vi "autoslice_delta_z_fixed.vi"() -> ()   [LabVIEW 2021]
panel:
  in  "Non moving mode":bool
  in  "System state during slices":string(combo)="Continuous imaging"
  in  "pulse duration (T/2)":dbl=0.0005 format="%#_13p"
  in  "Motor speed":string(combo)="Full step"
  in  "Use predefined list":bool
  in  "Predefined pulse steps":i32[](array[numeric])=[127, 63, 62, 58, 56, -72, -104, 24, 8, 72, 73, 77, 79, 15, 47, -81, -65, -97, 31, 29, 28, 92, 76, 12, 4, 36, -92, -90, -89, -121, -105, -41, -33, -49, -113, -114, 14, 46, 38, 6, 2, 18, 82, 83, -45, -61, -53, -21, -17, -25, -57, 71, 7, 23, 19, 3, 1, 9, 41, -87, -23, -31, -27, -11, -9, -13, -29, -93, -125, -117, -119, -127, -128, -124, -108, -44, -12, -16, -14, -6, -5, -7, -15, -47, -63, -59, -60, -64, 64, 66, 74, 106, 122, 120, 121, 125, -3, -4, -8, -24, -32, -30, 98, 96, 32, 33, 37, 53, 61, 60, -68, -66, -2, 126, 124, 116, 112, 113, 49, 48, 16, -112, -110, -102, -98, 30, 94, 95] format="%.0p"
  in  "milliseconds to wait after bed move":u32=500
  in  "milliseconds to wait after imaging ends":u32=500
  in  "pulses to move (delta z)":i32=20
  out "pulses moving":i32=20
  out "Wait for imaging":bool
  out "Wait for move":bool
  in  "max runs":i32=6 min=2 step=2
  out "Current run":i32=6
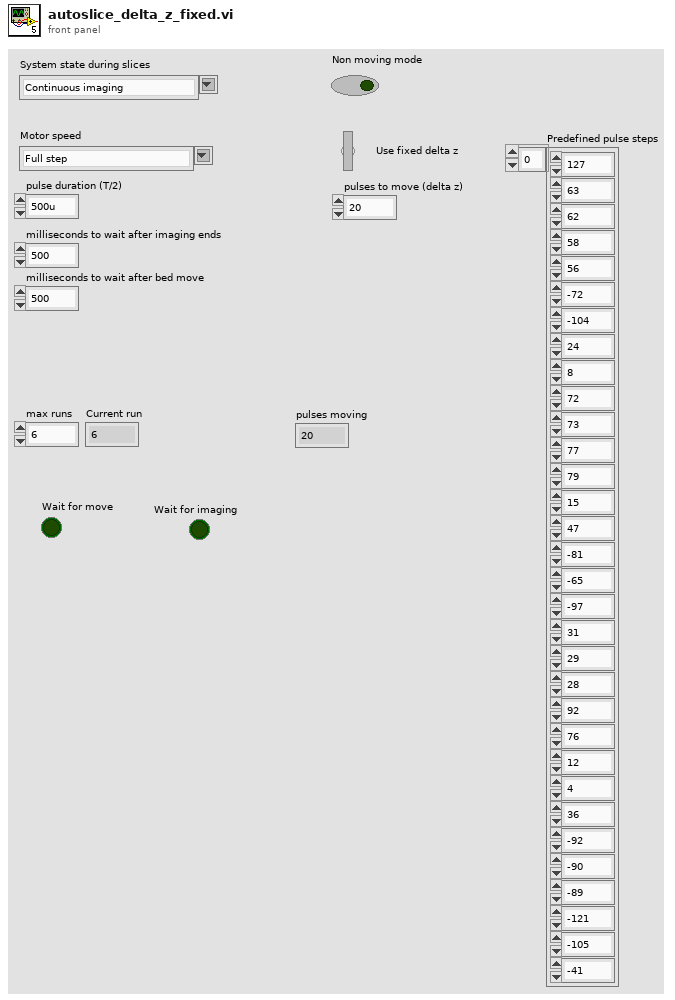
[diagram p1: front panel]
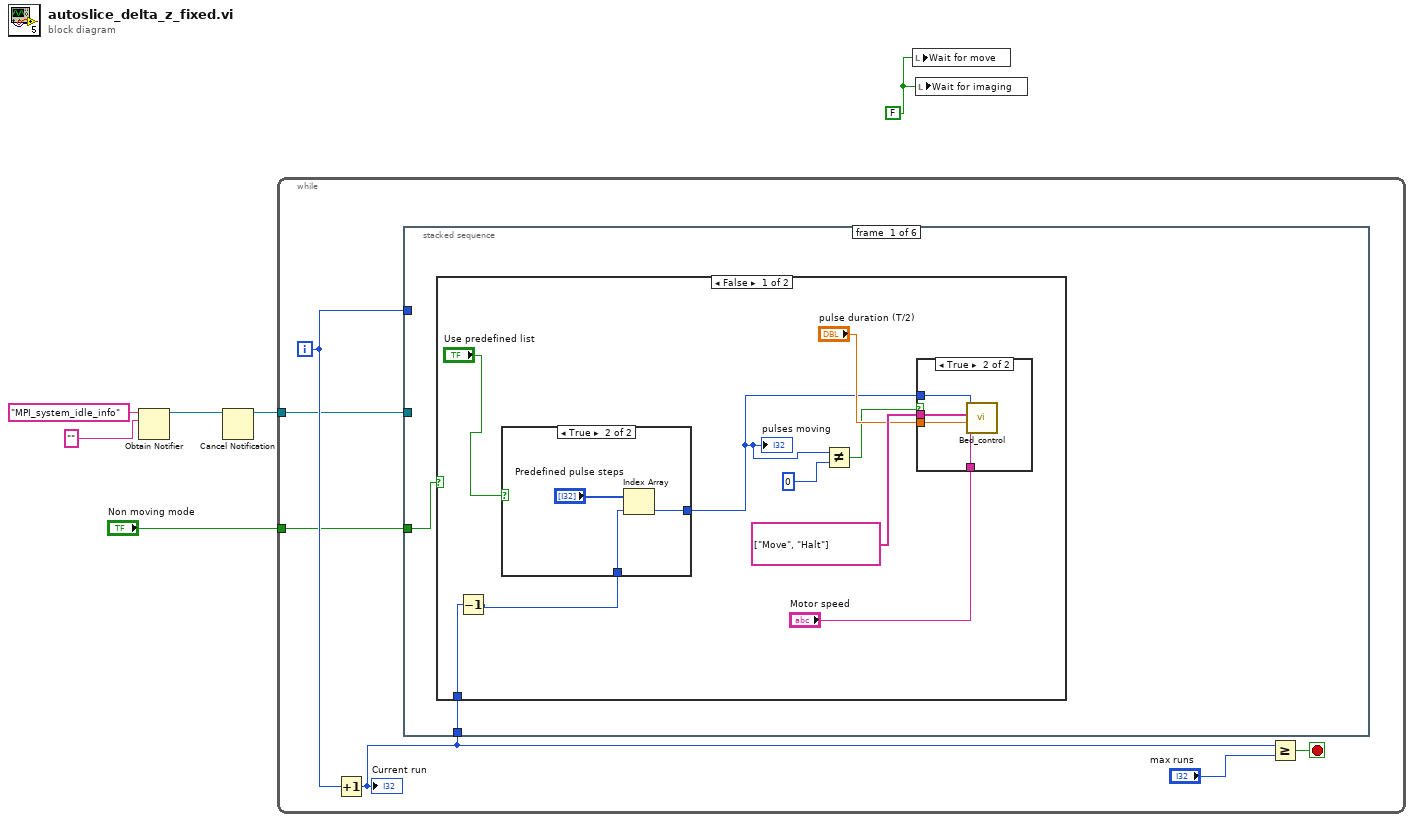
[diagram p0: block diagram]
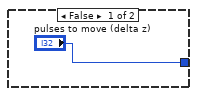
[diagram p3: hidden frame]
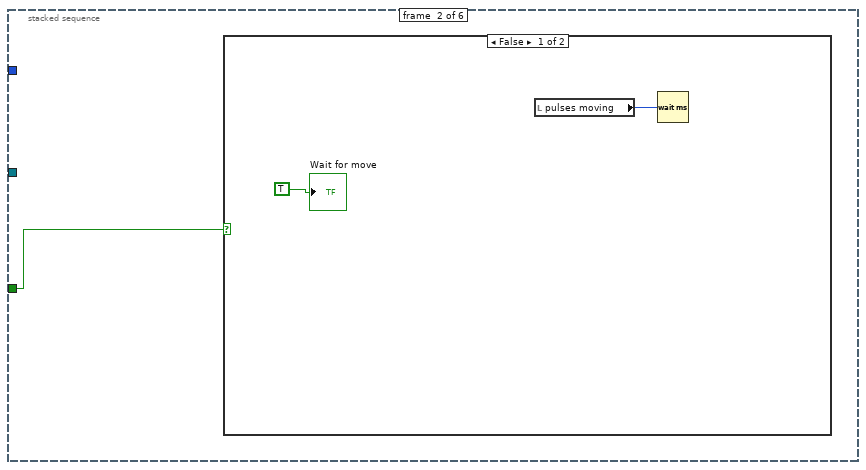
[diagram p5: hidden frame]
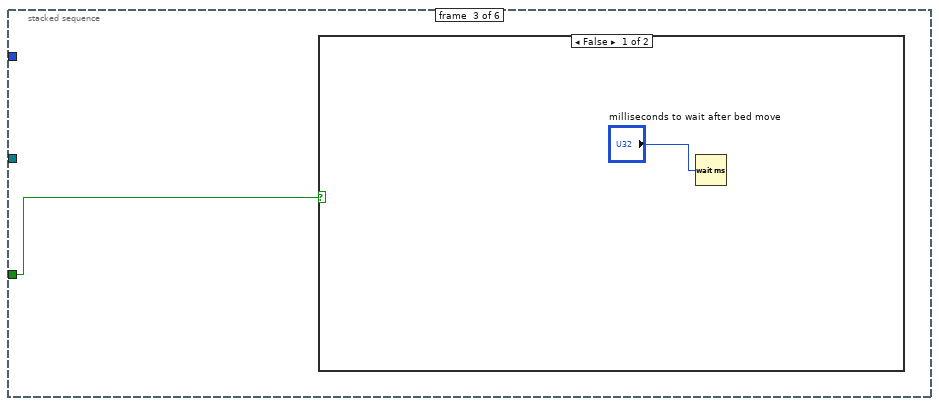
[diagram p7: hidden frame]
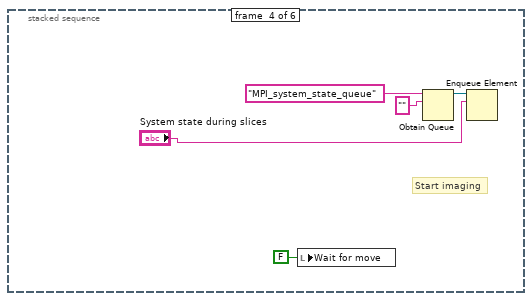
[diagram p9: hidden frame]
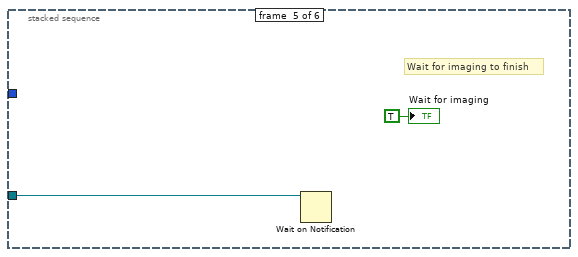
[diagram p10: hidden frame]
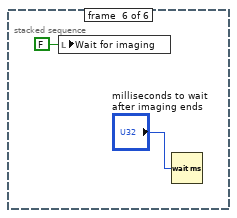
[diagram p11: hidden frame]
diagram:
  w2 = FALSE ("Boolean")
  n1 = Obtain Notifier(name (unnamed)="MPI_system_idle_info", notification data type="") -> (notifier out=w3:refnum<notifier>)  [unwired: 2 in, 2 out]
  n2 = Cancel Notification(0:w3) -> (8:w4:refnum<notifier>)  [unwired: 1 in, 2 out]
  n3 = while {
    tunnel: w4 -> [w9]
    tunnel: "Non moving mode" -> [w7]
    i -> [w10]
    stop <- w11 stop-if-true
    n4 = Increment(x=w10) -> (x+1=w8:i32)
    "Current run" <- w8
    n5 = stacked-sequence {
      tunnel: w10 -> [_ _ _ _ _ _]
      tunnel: w9 -> [_ _ _ _ w42 _]
      tunnel: w8 -> [w14 _ _ _ _ _]
      tunnel: w7 -> [w13 w32 w35 _ _ _]
      frame #0 {
        n6 = case shown="False" w13 {
          tunnel: w14 -> [w23 _]
          frame False {
            n7 = Decrement(x=w23) -> (x-1=w21:i32)
            n8 = case shown="True" "Use predefined list" {
              tunnel: w21 -> [_ w31]
              tunnel: ["pulses to move (delta z)" w29] -> w17
              frame False {
              }
              frame True {
                n9 = Index Array(array="Predefined pulse steps", index=w31) -> (element=w29:i32)
              }
            }
            "pulses moving" <- w17
            n10 = Not Equal?(x=w17, y=0) -> (x != y?=w15:bool)
            n11 = case shown="True" w15 {
              tunnel: string[] ["Move", "Halt"] ("Sequence to run on start up") -> [_ w27]
              tunnel: w17 -> [_ w26]
              tunnel: "Motor speed" -> [_ w25]
              tunnel: "pulse duration (T/2)" -> [_ w24]
              frame False {
              }
              frame True {
                n12 = call "Bed_control.vi"("Motor speed"=w25, "pulse duration (T/2)"=w24, "Sequence to run on start up"=w27, "Signed pulses to move"=w26) -> ()  [unwired: 8 in]
              }
            }
          }
          frame True {
          }
        }
      }
      frame #1 {
        n13 = case shown="False" w32 {
          frame False {
            n14 = local read "pulses moving"() -> (w33:i32)
            n15 = Wait (ms)(milliseconds to wait=w33) -> ()  [unwired: 1 out]
            "Wait for move" <- TRUE ("Wait for move")
          }
          frame True {
          }
        }
      }
      frame #2 {
        n16 = case shown="False" w35 {
          frame False {
            n17 = Wait (ms)(milliseconds to wait="milliseconds to wait after bed move") -> ()  [unwired: 1 out]
          }
          frame True {
          }
        }
      }
      frame #3 {
        # "Start imaging"
        n18 = local write "Wait for move"(FALSE ("Wait for move")) -> ()
        n19 = Obtain Queue(name (unnamed)="MPI_system_state_queue", element data type="" ("Type def")) -> (queue out=w41:refnum<queue>)  [unwired: 3 in, 2 out]
        n20 = Enqueue Element(queue=w41, element="System state during slices") -> ()  [unwired: 2 in, 3 out]
      }
      frame #4 {
        # "Wait for imaging to finish"
        n21 = Wait on Notification(notifier=w42) -> ()  [unwired: 3 in, 4 out]
        "Wait for imaging" <- TRUE ("Wait for imaging")
      }
      frame #5 {
        n22 = local write "Wait for imaging"(FALSE ("Wait for imaging")) -> ()
        n23 = Wait (ms)(milliseconds to wait="milliseconds to wait after imaging ends") -> ()  [unwired: 1 out]
      }
    }
    n24 = Greater Or Equal?(x=w8, y="max runs") -> (x >= y?=w11:bool)
  }
  n25 = local write "Wait for move"(w2) -> ()
  n26 = local write "Wait for imaging"(w2) -> ()
